vi "initialiseLasers.vi"(1 "642 nm":bool, 2 "561 nm":bool, 3 "488 nm":bool, 4 "405 nm":bool) -> (0 "initializedLasers":T1(array[cluster]))   [LabVIEW 2015]
uses:
  <vilib>/Instr/_visa.llb/VISA Configure Serial Port (Instr).vi
panel:
  in  "Laser comms":T2(array[cluster])=[{"baud rate "=500000, "data bits "=8, "parity "=enum."None", "flow control "=0, "timeout "=10000, "stop bits "=10}, {"baud rate "=57600, "data bits "=8, "parity "=enum."None", "flow control "=0, "timeout "=10000, "stop bits "=10}] {"stop bits" items=["1.0"=10, "1.5"=15, "2.0"=20]; "flow control" items=["None", "XON/XOFF", "RTS/CTS", "XON/XOFF & RTS/CTS", "DTR/DSR", "XON/XOFF & DTR/DSR"]}
  in  "LSFM_3 lasers":T1(array[cluster])=[{"Component ID"="405nm", "COM Port"="COM14", "Type "=enum."omicronLuxX", "init"=0}, {"Component ID"="488nm", "COM Port"="COM4", "Type "=enum."omicronLuxX", "init"=0}, {"Component ID"="561nm", "COM Port"="COM27", "Type "=enum."coherentObis", "init"=0}, {"Component ID"="642nm", "COM Port"="COM12", "Type "=enum."omicronLuxX", "init"=0}]
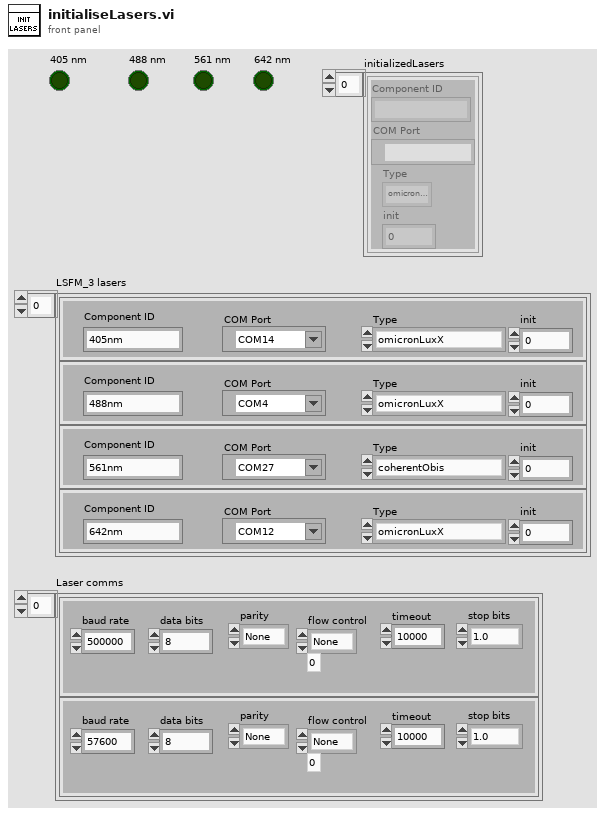
[diagram p1: front panel]
types:
  T1 = cluster{"Component ID":string, "COM Port":refnum<visa-resource-name>, "Type ":enum16{"omicronLuxX", "coherentObis"}, "init":i16}[]
  T2 = cluster{"baud rate ":u32, "data bits ":u16, "parity ":enum16{"None", "Odd", "Even", "Mark", "Space"}, "flow control ":u16, "timeout ":u32, "stop bits ":u16}[]
  T3 = cluster{"baud rate ":u32, "data bits ":u16, "parity ":enum16{"None", "Odd", "Even", "Mark", "Space"}, "flow control ":u16, "timeout ":u32, "stop bits ":u16}
  T4 = cluster{"Component ID":string, "COM Port":refnum<visa-resource-name>, "Type ":enum16{"omicronLuxX", "coherentObis"}, "init":i16}
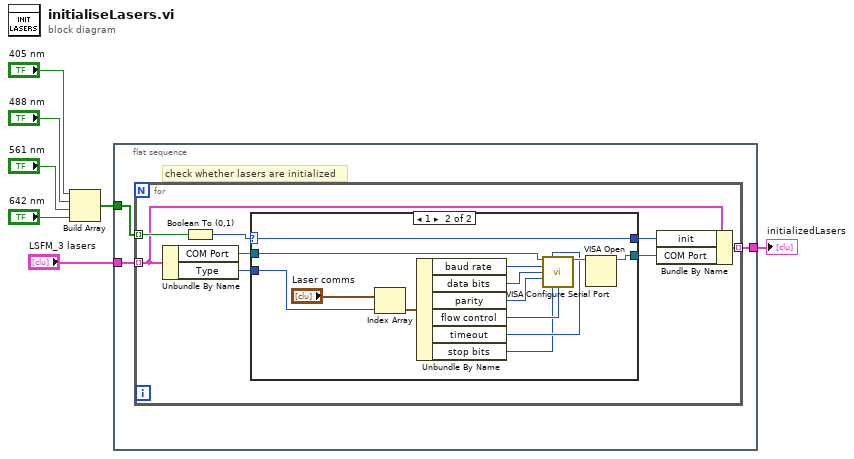
[diagram p0: block diagram]
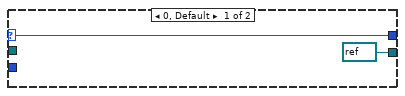
[diagram p2: hidden frame]
diagram:
  n1 = Build Array("405 nm", "488 nm", "561 nm", "642 nm") -> (w3:bool[])
  n2 = flat-sequence {
    tunnel: w3 -> [w10]
    tunnel: "LSFM_3 lasers" -> [w9]
    tunnel: [w8] -> w1
    frame #0 {
      # "check whether lasers are initialized"
      n3 = for {
        tunnel: w10 -> [w18] mode=indexing
        tunnel: w9 -> [w12] mode=indexing
        tunnel: [w11] -> w8 mode=indexing
        n4 = Unbundle By Name(w12) -> ("COM Port"=w15:refnum<visa-resource-name>, "Type"=w16:enum16{"omicronLuxX", "coherentObis"})
        n5 = Boolean To (0,1)(Boolean=w18) -> (0, 1=w17:i16)
        n6 = case shown="1" w17 {
          selector: w17 -> [w20 w21]
          tunnel: w16 -> [_ w26]
          tunnel: w15 -> [_ w23]
          tunnel: [refnum<visa-resource-name> refnum ("VISA resource name out") w22] -> w14
          tunnel: [w20 w21] -> w13
          frame 0, Default {
          }
          frame 1 {
            n7 = Index Array(array="Laser comms", index=w26) -> (element=w24:T3)
            n8 = Unbundle By Name(w24) -> ("baud rate"=w32:u32, "data bits"=w31:u16, "parity"=w30:enum16{"None", "Odd", "Even", "Mark", "Space"}, "flow control"=w29:u16, "timeout"=w28:u32, "stop bits"=w27:u16)
            n9 = call-poly "VISA Configure Serial Port"("VISA resource name"=w23, "timeout (10sec)"=w28, "baud rate (9600)"=w32, "data bits (8)"=w31, "parity (0:none)"=w30, "stop bits (10: 1 bit)"=w27, "flow control (0:none)"=w29) -> ("VISA resource name out"=w33:refnum<visa-resource-name>)  [unwired: 7 in, 1 out]
            n10 = VISA Open(VISA resource name=w33) -> (VISA resource name=w22:refnum<visa-resource-name>)  [unwired: 4 in, 1 out]
          }
        }
        n11 = Bundle By Name(cluster=w12, "init"=w13, "COM Port"=w14) -> (w11:T4)
      }
    }
  }
  "initializedLasers" <- w1
